vi "ISEG_HVChannel.createDIMservices.vi"(0 "i ref in":refnum<vi>, 5 "error in":errorcluster) -> (14 "i ref out":refnum<vi>, 19 "error out":errorcluster)   [LabVIEW 2014, in "ISEG_HVChannel.lvlib"]
doc: "creates the DIM service of some attributes"
uses:
  ISEG_HVChannel.lvlib
  CSlibraries-extern/DimLVEvent/LVDimInterface/LVDimInterface.lvlib
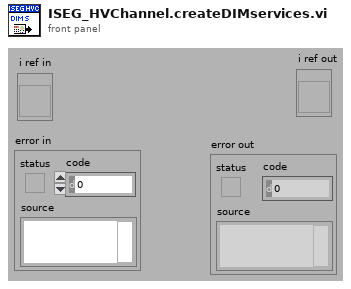
[diagram p1: front panel]
types:
  T1 = typedef "ISEG_HVChannel.lvlib/ISEG_HVChannel.i attribute.ctl" = cluster{"Channel Array":cluster{"Logical Name":string, "Address":string, "error in (no error)":errorcluster, "Status":cluster{"Status":i16, "DIM Status":T2}, "On":cluster{"On":bool, "DIM Status":T2}, "VMeas ":cluster{"VMeas":dbl, "DIM Status":T2}, "VSet ":cluster{"VSet":dbl, "DIM Status":T2}, "ITrip ":cluster{"ITrip":dbl, "DIM Status":T2}, "IMeas":cluster{"IMeas":dbl, "DIM Status":T2}, " RampSpeed":cluster{"RampSpeed":dbl, "DIM Status":T2}, "EventMask ":cluster{"EventMask":i16, "DIM Status":T2}}[], "VoltageInRangeBand":dbl, "NofCh":cluster{"NofCh":i32, "DIM Service":i32}, "BoardPrefix":string}
  T2 = typedef "ISEG_HVChannel.lvlib/ISEG_HVChannel.DIM Status.ctl" = cluster{"no link":bool, "quality":i32, "Time Stamp":timestamp}
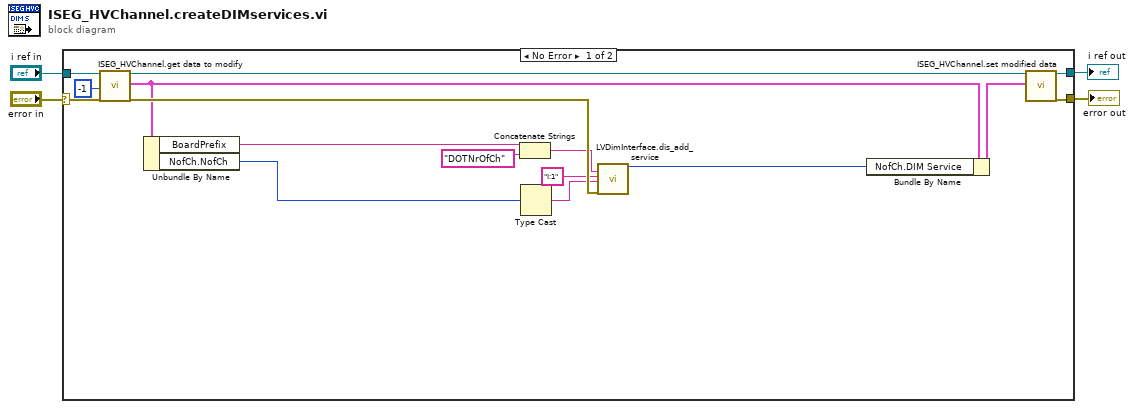
[diagram p0: block diagram]
diagram:
  n1 = case shown="No Error" "error in" {
    selector: "error in" -> [w19 w21]
    tunnel: "i ref in" -> [w20 w22]
    tunnel: [w16 w21] -> w3
    tunnel: [w17 w22] -> w2
    frame No Error {
      n2 = call "ISEG_HVChannel.get data to modify.vi"("i ref in"=w20, "ms timeout (10000)"=-1, "error in (no error)"=w19) -> ("i ref out"=w15:refnum<vi>, "i attribute"=w12:T1, "error out"=w14:errorcluster)  [unwired: 13 in, 1 out]
      n3 = Unbundle By Name(w12) -> ("BoardPrefix"=w5:string, "NofCh.NofCh"=w10:i32)
      n4 = Concatenate Strings(w5, "DOTNrOfCh" ("string")) -> (w7:string)
      n5 = Type Cast(x=w10) -> (*(type *) &x=w6:string)  [unwired: 1 in]
      n6 = call "LVDimInterface.dis_add_service.vi"("serviceName"=w7, "typeDescriptor"="I:1", "data"=w6, "error in (no error)"=w14) -> ("my_serviceID"=w9:i32)  [unwired: 14 in, 1 out]
      n7 = Bundle By Name(cluster=w12, "NofCh.DIM Service"=w9) -> (w13:T1)
      n8 = call "ISEG_HVChannel.set modified data.vi"("i ref in"=w15, "i attribute"=w13) -> ("i ref out"=w17:refnum<vi>, "error out"=w16:errorcluster)  [unwired: 16 in]
    }
    frame Error {
    }
  }
  "i ref out" <- w2
  "error out" <- w3
